vi "Function Generator.vi"(11 "Properties in":T1={"Schedule"=0, "Value"=0.0, "Start Value"=0.0, "End Value"=0.0, "Min Value"=0.0, "Max Value"=0.0, "Duty Cycle (%)"=0.0, "Speed Signal Type"=2, "Cycle Number"=0.0, "Phase (degrees)"=0.0} {"Schedule" items=["Constant", "Ramp", "Fn. Generator", "Formula"]; "Speed Signal Type" items=["Sine Wave", "Triangle Wave", "Square Wave", "Sawtooth Wave"]}) -> (2 "Properties out":T1={"Schedule"=0, "Value"=0.0, "Start Value"=0.0, "End Value"=0.0, "Min Value"=1.0, "Max Value"=3.0, "Duty Cycle (%)"=56.0, "Speed Signal Type"=0, "Cycle Number"=3.0, "Phase (degrees)"=90.0} {"Schedule" items=["Constant", "Ramp", "Fn. Generator", "Formula"]; "Speed Signal Type" items=["Sine Wave", "Triangle Wave", "Square Wave", "Sawtooth Wave"]}, 3 "Cancelled?":bool)   [LabVIEW 2013]
doc: "Use this template to create a dialog box with event handling."
uses:
  <vilib>/measure/NI_MABase.lvlib
panel:
  in  "Samples (testing)":dbl=1000.0
  out "Signal":dbl[](graph)=[3.0, 2.999822352380809, 2.999289472640589, 2.998401550108975, 2.997158900260614, 2.99556196460308, 2.9936113105200084, 2.991307631069507, 2.988651744737914, 2.9856445951489983, 2.982287250728689, 2.9785809043254723, 2.9745268727865772, 2.970126596490106, 2.965381638833274, 2.960293685676943, 2.954864544746643, 2.9490961449902944, 2.9429905358928643, 2.9365498867481925, 2.9297764858882513, 2.922672739870115, 2.9152411726209175, 2.907484424541117, 2.899405251566371, 2.891006524188368, 2.882291226434953, 2.87326245480992, 2.863923417192835, 2.854277431699295, 2.844327925502015, 2.834078433613171, 2.8235325976284273, 2.812694164433094, 2.8015669848708766, 2.79015501237569, 2.778462301567023, 2.76649300680935, 2.754251380736104, 2.741741772738739, 2.7289686274214113, 2.715936483021831, 2.7026499697988493, 2.6891138083873485, 2.6753328081210244, 2.661311865323652, 2.6470559615694444, 2.6325701619131245, 2.617859613090334, 2.602929541689025, 2.587785252292473, 2.572432125594591, 2.556875616488188, 2.5411212521268762, 2.525174629961296, 2.5090414157503713, 2.4927273415482913, 2.4762382036679393, 2.459579860621488, 2.4427582310389018, 2.425779291565073, 2.408649074736349, 2.3913736668372025, 2.3739592057378007, 2.3564118787132506, 2.3387379202452916, 2.3209436098072094, 2.3030352696327743, 2.285019262469976, 2.2669019893203757, 2.248689887164855, 2.2303894266765907, 2.212007109922055, 2.1935494680508603, 2.175023058975276, 2.156434465040231, 2.137790290684638, 2.11909716009487, 2.100361714851215, 2.0815906115681577, 2.0627905195293135, 2.0439681183178653, 2.0251300954433376, 2.0062831439655593, 1.9874339601166475, 1.968589240921872, 1.9497556818202306, 1.9309399742855944, 1.912148803449257, 1.8933888457247403, 1.874666766435696, 1.855989217447748, 1.8373628348051165, 1.8187942363728629, 1.800290019485593, 1.7818567586034577, 1.7635010029762754, 1.745229274316618, 1.727048064482675, 1.7089638331717283, 1.6909830056250528, 1.6731119703450577, 1.6553570768254833, 1.6377246332954545, 1.6202209044781992, 1.6028521093652195, 1.5856244190067161, 1.5685439543190411, 1.551616783909968, 1.5348489219225419, 1.518246325898285, 1.5018148946605094, 1.4855604662184938, 1.4694888156932662, 1.4536056532657313, 1.4379166221478696, 1.4224272965777327, 1.407143179838941, 1.392069702305395, 1.3772122195118879, 1.3625760102513107, 1.3481662746991216, 1.3339881325657488, 1.320046621277581, 1.3063466941871953, 1.2928932188134528, 1.2796909751120933, 1.2667446537774403, 1.2540588545758182, 1.2416380847112785, 1.229486757224211, 1.217609189423412, 1.2060096013521648, 1.1946921142888782, 1.1836607492828162, 1.1729194257254383, 1.1624719599578586, 1.152322063914917, 1.142473343806348, 1.1329292988355102, 1.1236933199561365, 1.114768688667545, 1.1061585758487364, 1.0978660406317973, 1.0898940293150043, 1.082245374316019, 1.074922793165542, 1.0679288875417892, 1.061266142346126, 1.0549369248201954, 1.0489434837048466, 1.04328794844117, 1.0379723284139142, 1.0329985122375653, 1.0283682670853262, 1.024083238061253, 1.0201449476157534, 1.0165547950046707, 1.013314055792132, 1.0104238813973492, 1.0078852986855225, 1.0056992096030013, 1.0038663908568277, 1.0023874936387749, 1.0012630433939829, 1.0004934396342686, 1.0000789557961842, 1.000019739143863, 1.0003158107167003, 1.0009670653218754, 1.0019732715717287, 1.0033340719659702, 1.0050489830187002, 1.0071173954301864, 1.009538574303349, 1.0123116594048622, 1.0154356654707948, 1.018909482556666, 1.0227318764318067, 1.0269014890178734, 1.031416838871369, 1.0362763217099902, 1.0414782109826244, 1.047020658482781, 1.0529016950052559, 1.0591192310457744, 1.065671057543388, 1.0725548466653385, 1.0797681526341298, 1.0873084125964971, 1.0951729475339806, 1.103358963214764, 1.1118635511864556, 1.1206836898094434, 1.1298162453304745, 1.139257972996056, 1.1490055182053083, 1.1590554177018304, 1.1694041008041873, 1.1800478906745473, 1.1909830056250525, 1.2022055604614286, 1.2137115678633812, 1.2254969398012658, 1.2375574889885521, 1.24988893036954, 1.2624868826418263, 1.2753468698129529, 1.2884643227907149, 1.3018345810065268, 1.3154528940713113, 1.3293144234632794, 1.3434142442470436, 1.3577473468234151, 1.3723086387092995, 1.387092946347023, 1.4020950169424813, 1.4173095203314234, 1.4327310508732436, 1.4483541293715692, 1.4641732050210035, 1.48018265737929, 1.4963767983642393, 1.5127498742746672, 1.5292960678346674, 1.5460095002604528, 1.5628842333490671, 1.5799142715881933, 1.5970935642863373, 1.6144160077226029, 1.631875447315322, 1.6494656798087406, 1.6671804554770133, 1.6850134803446948, 1.702958418422965, 1.7210088939607702, 1.739158493710103, 1.757400769204592, 1.7757292390506187, 1.7941373912301182, 1.8126186854142752, 1.8311665552872656, 1.8497744108792429, 1.868435640907717, 1.8871436151265182, 1.9058916866814852, 1.9246731944720672, 1.9434814655179748, 1.9623098173300653, 1.9811515602845913, 1.9999999999999998, 2.018848439715408, 2.0376901826699343, 2.056518534482024, 2.0753268055279324, 2.0941083133185137, 2.1128563848734814, 2.131564359092282, 2.150225589120757, 2.1688334447127335, 2.1873813145857244, 2.205862608769881, 2.224270760949381, 2.242599230795407, 2.2608415062898968, 2.2789911060392285, 2.2970415815770346, 2.3149865196553043, 2.3328195445229865, 2.3505343201912585, 2.3681245526846775, 2.385583992277396, 2.4029064357136622, 2.420085728411806, 2.4371157666509324, 2.4539904997395463, 2.4707039321653324, 2.487250125725332, 2.5036232016357607, 2.519817342620709, 2.535826794978996, 2.5516458706284295, 2.567268949126756, 2.5826904796685755, 2.5979049830575187, 2.612907053652976, 2.6276913612907, 2.642252653176584, 2.656585755752956, 2.6706855765367195, 2.6845471059286883, 2.6981654189934723, 2.7115356772092847, 2.724653130187046, 2.7375131173581737, 2.750111069630459, 2.7624425110114474, 2.7745030601987333, 2.7862884321366184, 2.7977944395385705, 2.809016994374947, 2.819952109325452, 2.8305958991958122, 2.8409445822981687, 2.8509944817946913, 2.860742027003943, 2.870183754669525, 2.879316310190556, 2.888136448813544, 2.8966410367852355, 2.904827052466019, 2.9126915874035024, 2.92023184736587, 2.927445153334661, 2.9343289424566117, 2.9408807689542256, 2.9470983049947437, 2.952979341517219, 2.9585217890173756, 2.96372367829001, 2.9685831611286306, 2.9730985109821266, 2.977268123568193, 2.9810905174433344, 2.984564334529205, 2.9876883405951378, 2.990461425696651, 2.9928826045698136, 2.9949510169813, 2.99666592803403, 2.9980267284282713, 2.999032934678125, 2.9996841892832995, 2.9999802608561374, 2.999921044203816, 2.999506560365732, 2.998736956606017, 2.9976125063612256, 2.996133609143172, 2.9943007903969994, 2.9921147013144775, 2.9895761186026513, 2.986685944207868, 2.9834452049953297, 2.9798550523842464, 2.9759167619387474, 2.9716317329146738, 2.9670014877624356, 2.9620276715860854, 2.9567120515588305, 2.951056516295153, 2.9450630751798053, 2.9387338576538737, 2.9320711124582113, 2.925077206834458, 2.9177546256839815, 2.910105970684995, 2.902133959368203, 2.8938414241512636, 2.8852313113324555, 2.8763066800438635, 2.8670707011644905, 2.8575266561936523, 2.8476779360850837, 2.8375280400421414, 2.827080574274562, 2.816339250717184, 2.805307885711122, 2.793990398647835, 2.7823908105765884, 2.770513242775789, 2.7583619152887224, 2.745941145424182, 2.7332553462225606, 2.720309024887907, 2.707106781186548, 2.693653305812805, 2.67995337872242, 2.6660118674342517, 2.6518337253008792, 2.6374239897486897, 2.622787780488113, 2.6079302976946055, 2.59285682016106, 2.577572703422268, 2.5620833778521312, 2.546394346734269, 2.530511184306735, 2.5144395337815064, 2.4981851053394917, 2.4817536741017157, 2.465151078077459, 2.4483832160900327, 2.4314560456809597, 2.4143755809932843, 2.3971478906347814, 2.3797790955218012, 2.362275366704546, 2.344642923174517, 2.3268880296549432, 2.309016994374948, 2.2910361668282726, 2.2729519355173258, 2.254770725683383, 2.236498997023725, 2.218143241396543, 2.1997099805144074, 2.1812057636271382, 2.162637165194884, 2.144010782552253, 2.1253332335643047, 2.1066111542752606, 2.0878511965507434, 2.0690600257144065, 2.05024431817977, 2.031410759078129, 2.012566039883353, 1.9937168560344418, 1.974869904556663, 1.9560318816821358, 1.937209480470687, 1.9184093884318432, 1.8996382851487856, 1.8809028399051309, 1.8622097093153624, 1.8435655349597697, 1.8249769410247245, 1.8064505319491404, 1.7879928900779458, 1.7696105733234102, 1.7513101128351458, 1.7330980106796252, 1.7149807375300243, 1.6969647303672266, 1.679056390192791, 1.6612620797547093, 1.6435881212867498, 1.6260407942622002, 1.6086263331627981, 1.5913509252636515, 1.5742207084349278, 1.5572417689610991, 1.5404201393785126, 1.5237617963320613, 1.5072726584517089, 1.4909585842496291, 1.4748253700387048, 1.4588787478731247, 1.4431243835118126, 1.4275678744054094, 1.4122147477075275, 1.3970704583109756, 1.3821403869096662, 1.367429838086876, 1.3529440384305562, 1.3386881346763486, 1.324667191878976, 1.310886191612652, 1.2973500302011514, 1.2840635169781691, 1.2710313725785891, 1.258258227261261, 1.2457486192638967, 1.2335069931906504, 1.221537698432977, 1.2098449876243098, 1.1984330151291238, 1.1873058355669062, 1.176467402371573, 1.165921566386829, 1.1556720744979856, 1.1457225683007048, 1.1360765828071653, 1.1267375451900798, 1.1177087735650473, 1.1089934758116322, 1.1005947484336294, 1.092515575458883, 1.084758827379083, 1.0773272601298851, 1.070223514111749, 1.0634501132518075, 1.0570094641071361, 1.0509038550097052, 1.0451354552533574, 1.0397063143230567, 1.0346183611667266, 1.029873403509894, 1.0254731272134232, 1.0214190956745277, 1.0177127492713116, 1.0143554048510017, 1.0113482552620865, 1.0086923689304932, 1.006388689479992, 1.0044380353969196, 1.0028410997393864, 1.0015984498910246, 1.000710527359411, 1.0001776476191906, 1.0000000000000002, 1.0001776476191906, 1.000710527359411, 1.0015984498910246, 1.0028410997393862, 1.0044380353969196, 1.0063886894799916, 1.0086923689304932, 1.011348255262086, 1.0143554048510017, 1.0177127492713114, 1.0214190956745275, 1.0254731272134228, 1.0298734035098938, 1.0346183611667261, 1.0397063143230565, 1.045135455253357, 1.050903855009705, 1.0570094641071355, 1.063450113251807, 1.0702235141117487, 1.0773272601298847, 1.0847588273790825, 1.0925155754588824, 1.100594748433629, 1.1089934758116318, 1.1177087735650466, 1.1267375451900792, 1.1360765828071644, 1.1457225683007044, 1.1556720744979847, 1.1659215663868283, 1.1764674023715722, 1.1873058355669055, 1.198433015129123, 1.209844987624309, 1.2215376984329762, 1.2335069931906495, 1.2457486192638958, 1.2582582272612601, 1.2710313725785882, 1.284063516978168, 1.2973500302011503, 1.3108861916126509, 1.3246671918789752, 1.3386881346763473, 1.352944038430555, 1.3674298380868748, 1.3821403869096651, 1.3970704583109745, 1.4122147477075262, 1.4275678744054083, 1.4431243835118113, 1.4588787478731233, 1.4748253700387037, 1.4909585842496278, 1.5072726584517078, 1.5237617963320602, 1.5404201393785115, 1.5572417689610978, 1.5742207084349267, 1.5913509252636502, 1.608626333162797, 1.6260407942621988, 1.6435881212867485, 1.6612620797547077, 1.6790563901927897, 1.6969647303672253, 1.7149807375300232, 1.7330980106796237, 1.7513101128351445, 1.7696105733234087, 1.7879928900779447, 1.8064505319491388, 1.8249769410247232, 1.8435655349597684, 1.8622097093153611, 1.8809028399051295, 1.8996382851487843, 1.9184093884318416, 1.9372094804706859, 1.9560318816821343, 1.9748699045566618, 1.9937168560344403, 2.012566039883352, 2.0314107590781276, 2.050244318179769, 2.069060025714405, 2.0878511965507425, 2.1066111542752592, 2.1253332335643034, 2.1440107825522516, 2.162637165194883, 2.1812057636271365, 2.1997099805144065, 2.218143241396542, 2.236498997023724, 2.2547707256833815, 2.2729519355173244, 2.2910361668282713, 2.3090169943749466, 2.326888029654942, 2.3446429231745163, 2.362275366704545, 2.3797790955218003, 2.39714789063478, 2.4143755809932834, 2.4314560456809584, 2.448383216090032, 2.465151078077458, 2.4817536741017148, 2.4981851053394903, 2.514439533781506, 2.5305111843067336, 2.5463943467342687, 2.56208337785213, 2.577572703422267, 2.5928568201610585, 2.607930297694605, 2.622787780488112, 2.6374239897486893, 2.6518337253008784, 2.6660118674342512, 2.6799533787224186, 2.6936533058128047, 2.707106781186547, 2.7203090248879063, 2.7332553462225597, 2.7459411454241818, 2.758361915288721, 2.770513242775789, 2.7823908105765875, 2.793990398647835, 2.8053078857111213, 2.8163392507171836, 2.8270805742745617, 2.8375280400421414, 2.847677936085083, 2.8575266561936523, 2.86707070116449, 2.8763066800438635, 2.885231311332455, 2.8938414241512636, 2.9021339593682027, 2.9101059706849957, 2.917754625683981, 2.925077206834458, 2.932071112458211, 2.938733857653874, 2.945063075179805, 2.9510565162951536, 2.9567120515588305, 2.962027671586086, 2.967001487762435, 2.9716317329146738, 2.9759167619387474, 2.979855052384247, 2.9834452049953297, 2.986685944207868, 2.989576118602651, 2.9921147013144775, 2.994300790396999, 2.9961336091431723, 2.997612506361225, 2.9987369566060176, 2.999506560365732, 2.9999210442038162, 2.9999802608561374, 2.9996841892833, 2.999032934678125, 2.998026728428272, 2.99666592803403, 2.9949510169813003, 2.992882604569814, 2.9904614256966515, 2.987688340595138, 2.9845643345292054, 2.9810905174433344, 2.9772681235681935, 2.973098510982127, 2.9685831611286315, 2.9637236782900103, 2.958521789017376, 2.9529793415172194, 2.9470983049947446, 2.940880768954226, 2.934328942456612, 2.927445153334662, 2.9202318473658706, 2.9126915874035033, 2.90482705246602, 2.8966410367852364, 2.888136448813545, 2.879316310190557, 2.870183754669526, 2.8607420270039445, 2.850994481794692, 2.84094458229817, 2.830595899195813, 2.8199521093254534, 2.809016994374948, 2.797794439538572, 2.7862884321366197, 2.774503060198735, 2.7624425110114483, 2.7501110696304605, 2.7375131173581746, 2.724653130187048, 2.711535677209286, 2.6981654189934736, 2.684547105928689, 2.6706855765367212, 2.656585755752957, 2.6422526531765853, 2.627691361290701, 2.6129070536529775, 2.5979049830575196, 2.5826904796685772, 2.567268949126757, 2.5516458706284313, 2.5358267949789974, 2.5198173426207107, 2.5036232016357616, 2.4872501257253337, 2.4707039321653332, 2.453990499739548, 2.4371157666509338, 2.4200857284118076, 2.4029064357136636, 2.3855839922773976, 2.368124552684679, 2.3505343201912603, 2.3328195445229873, 2.314986519655306, 2.2970415815770355, 2.2789911060392303, 2.2608415062898977, 2.242599230795409, 2.224270760949382, 2.2058626087698827, 2.1873813145857257, 2.1688334447127353, 2.150225589120758, 2.131564359092284, 2.1128563848734827, 2.0941083133185154, 2.0753268055279337, 2.056518534482026, 2.0376901826699356, 2.0188484397154096, 2.000000000000001, 1.981151560284593, 1.9623098173300664, 1.9434814655179766, 1.924673194472068, 1.9058916866814868, 1.887143615126519, 1.8684356409077187, 1.8497744108792438, 1.8311665552872674, 1.8126186854142763, 1.7941373912301197, 1.7757292390506196, 1.7574007692045936, 1.739158493710104, 1.721008893960772, 1.7029584184229658, 1.6850134803446963, 1.6671804554770142, 1.649465679808742, 1.6318754473153227, 1.6144160077226044, 1.5970935642863382, 1.5799142715881946, 1.5628842333490678, 1.5460095002604541, 1.529296067834668, 1.5127498742746686, 1.4963767983642398, 1.4801826573792916, 1.4641732050210041, 1.4483541293715707, 1.4327310508732443, 1.417309520331425, 1.4020950169424817, 1.3870929463470243, 1.3723086387093002, 1.3577473468234165, 1.3434142442470443, 1.3293144234632808, 1.315452894071312, 1.3018345810065282, 1.2884643227907153, 1.275346869812954, 1.2624868826418267, 1.2498889303695413, 1.2375574889885526, 1.2254969398012667, 1.2137115678633816, 1.2022055604614295, 1.190983005625053, 1.1800478906745482, 1.1694041008041878, 1.1590554177018313, 1.1490055182053087, 1.1392579729960568, 1.1298162453304748, 1.120683689809444, 1.1118635511864559, 1.1033589632147645, 1.0951729475339809, 1.0873084125964976, 1.07976815263413, 1.072554846665339, 1.0656710575433883, 1.0591192310457749, 1.0529016950052559, 1.0470206584827815, 1.0414782109826244, 1.0362763217099904, 1.0314168388713691, 1.0269014890178734, 1.0227318764318067, 1.018909482556666, 1.0154356654707948, 1.0123116594048622, 1.009538574303349, 1.0071173954301862, 1.0050489830187, 1.0033340719659698, 1.0019732715717284, 1.000967065321875, 1.0003158107167, 1.0000197391438626, 1.0000789557961838, 1.0004934396342682, 1.0012630433939824, 1.0023874936387744, 1.0038663908568273, 1.0056992096030006, 1.007885298685522, 1.0104238813973485, 1.0133140557921316, 1.0165547950046698, 1.0201449476157527, 1.0240832380612521, 1.0283682670853258, 1.0329985122375644, 1.0379723284139137, 1.043287948441169, 1.048943483704846, 1.0549369248201945, 1.0612661423461254, 1.0679288875417883, 1.0749227931655416, 1.082245374316018, 1.089894029315004, 1.0978660406317964, 1.1061585758487356, 1.114768688667544, 1.1236933199561359, 1.132929298835509, 1.1424733438063472, 1.1523220639149159, 1.1624719599578577, 1.1729194257254374, 1.1836607492828155, 1.1946921142888773, 1.206009601352164, 1.2176091894234111, 1.22948675722421, 1.2416380847112771, 1.254058854575817, 1.266744653777439, 1.2796909751120922, 1.2928932188134517, 1.306346694187194, 1.3200466212775799, 1.3339881325657474, 1.3481662746991203, 1.3625760102513094, 1.3772122195118865, 1.3920697023053936, 1.4071431798389398, 1.4224272965777314, 1.4379166221478683, 1.45360565326573, 1.469488815693265, 1.4855604662184925, 1.501814894660508, 1.5182463258982837, 1.5348489219225407, 1.5516167839099666, 1.56854395431904, 1.5856244190067148, 1.6028521093652184, 1.6202209044781977, 1.6377246332954531, 1.6553570768254817, 1.6731119703450563, 1.6909830056250514, 1.708963833171727, 1.7270480644826736, 1.7452292743166167, 1.763501002976274, 1.7818567586034564, 1.8002900194855918, 1.8187942363728615, 1.8373628348051152, 1.8559892174477466, 1.8746667664356944, 1.8933888457247388, 1.9121488034492555, 1.930939974285593, 1.9497556818202293, 1.9685892409218704, 1.9874339601166462, 2.0062831439655575, 2.025130095443336, 2.0439681183178635, 2.062790519529312, 2.0815906115681564, 2.1003617148512137, 2.1190971600948685, 2.1377902906846367, 2.1564344650402294, 2.175023058975275, 2.193549468050859, 2.2120071099220535, 2.2303894266765893, 2.2486898871648537, 2.2669019893203743, 2.2850192624699748, 2.3030352696327725, 2.3209436098072085, 2.3387379202452903, 2.3564118787132498, 2.3739592057377994, 2.391373666837201, 2.408649074736348, 2.4257792915650715, 2.4427582310389004, 2.4595798606214867, 2.476238203667938, 2.4927273415482905, 2.50904141575037, 2.5251746299612945, 2.541121252126875, 2.556875616488187, 2.57243212559459, 2.5877852522924725, 2.602929541689024, 2.6178596130903333, 2.632570161913123, 2.6470559615694436, 2.661311865323651, 2.6753328081210235, 2.6891138083873476, 2.7026499697988484, 2.71593648302183, 2.728968627421411, 2.741741772738738, 2.754251380736103, 2.766493006809349, 2.778462301567023, 2.7901550123756893, 2.801566984870876, 2.8126941644330934, 2.823532597628427, 2.8340784336131706, 2.844327925502015, 2.8542774316992947, 2.863923417192835, 2.8732624548099195, 2.882291226434953, 2.8910065241883673, 2.899405251566371, 2.907484424541116, 2.9152411726209175, 2.922672739870114, 2.9297764858882513, 2.9365498867481916, 2.9429905358928643, 2.949096144990294, 2.954864544746643, 2.960293685676943, 2.965381638833274, 2.9701265964901054, 2.9745268727865772, 2.978580904325472, 2.982287250728689, 2.985644595148998, 2.988651744737914, 2.9913076310695064, 2.9936113105200084, 2.9955619646030796, 2.9971589002606143, 2.9984015501089747, 2.9992894726405894, 2.999822352380809]
  in  "Signal Type":u16(ring) items=["Sine Wave", "Triangle Wave", "Square Wave", "Sawtooth Wave"]
  in  "Phase (degrees)":dbl=90.0
  in  "Cycle Number":dbl=3.0
  in  "Square Wave\nDuty Cycle (%)":dbl=56.0
  in  "Max Value":dbl=3.0
  in  "Min Value":dbl=1.0
  in  "Cancel":bool
  in  "OK":bool
  # "Function Generator"
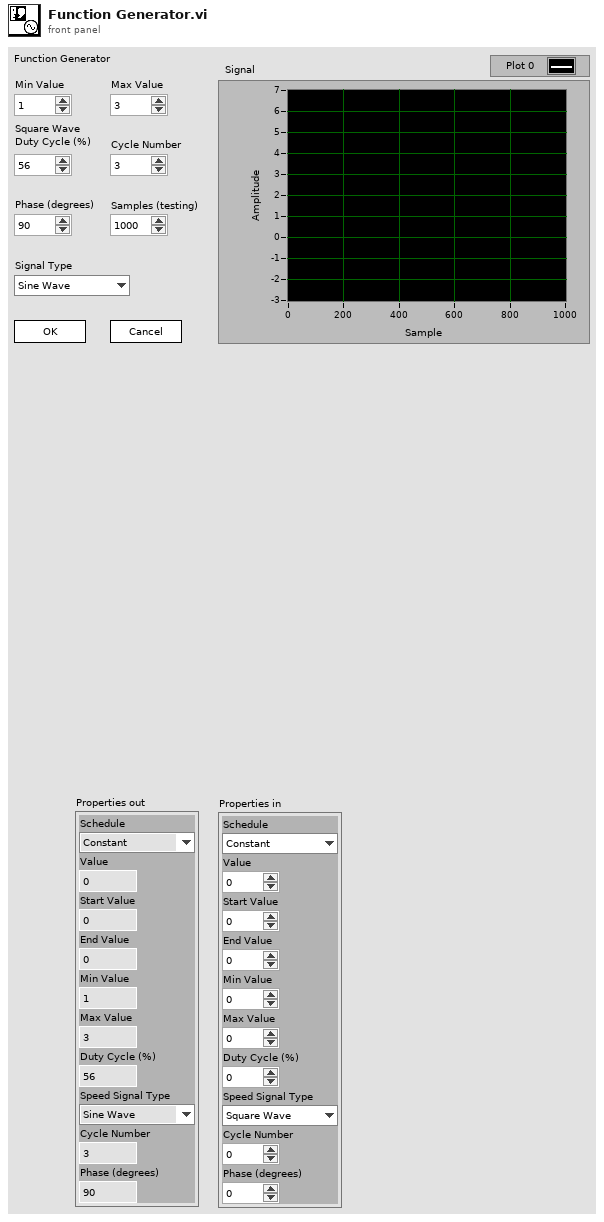
[diagram p1: front panel]
types:
  T1 = cluster{"Schedule":u16, "Value":dbl, "Start Value":dbl, "End Value":dbl, "Min Value":dbl, "Max Value":dbl, "Duty Cycle (%)":dbl, "Speed Signal Type":u16, "Cycle Number":dbl, "Phase (degrees)":dbl}
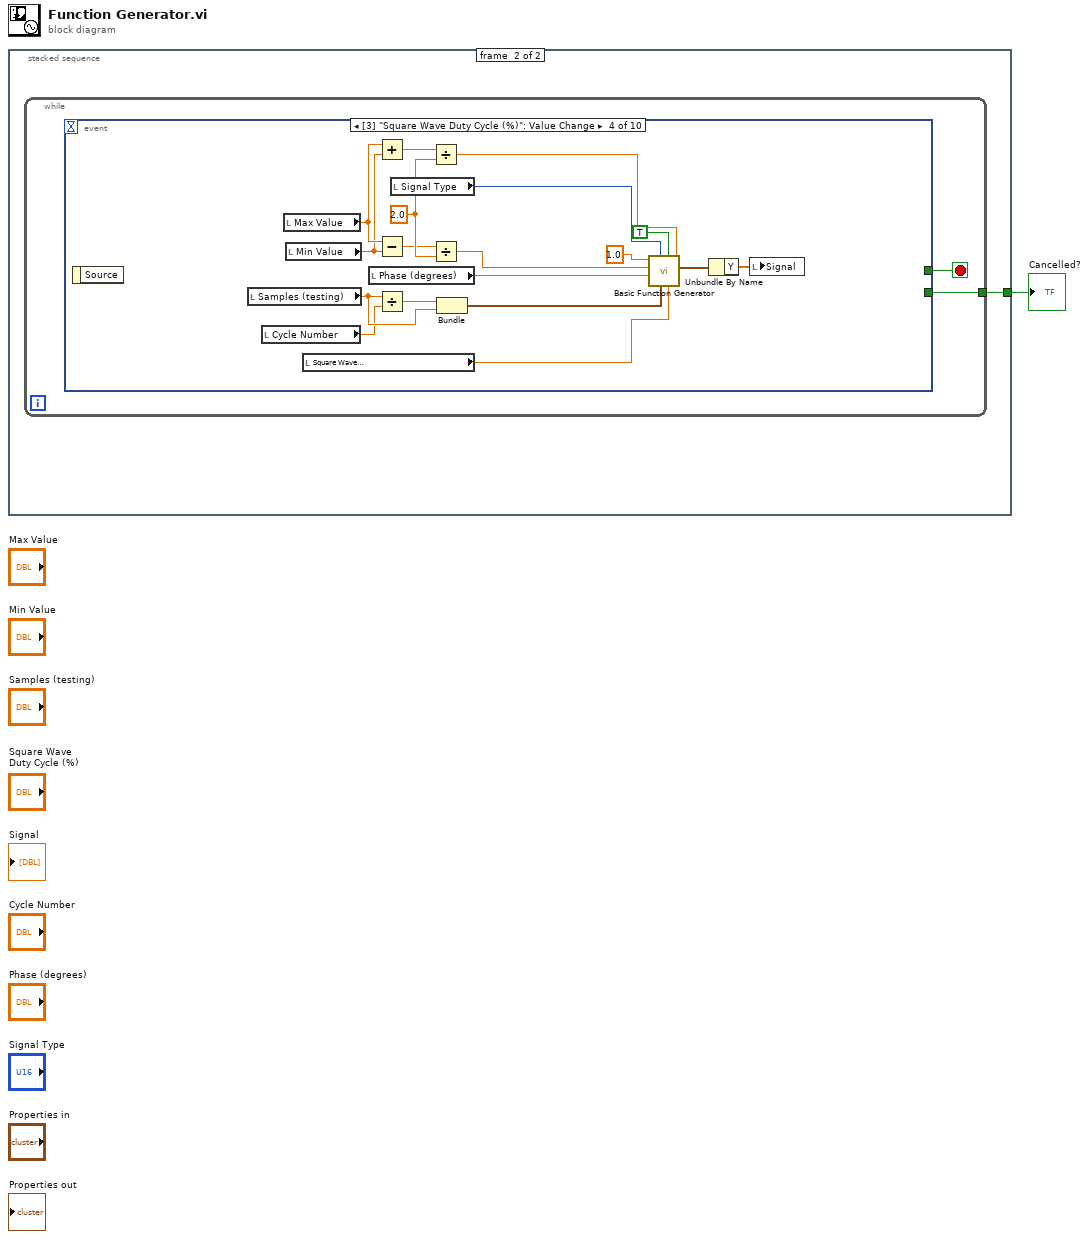
[diagram p0: block diagram]
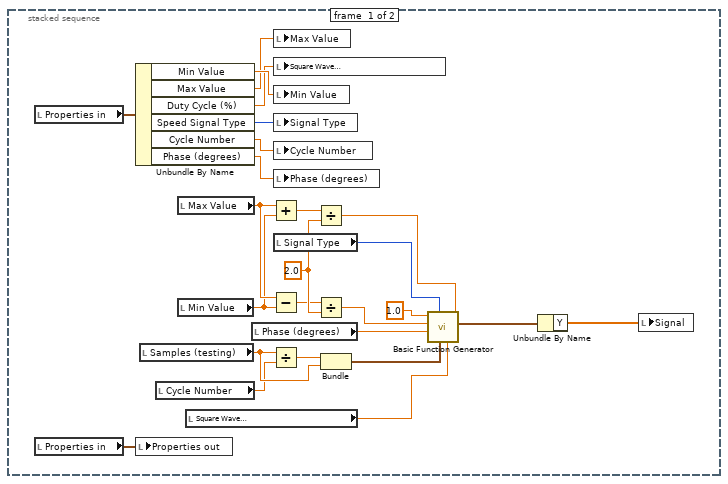
[diagram p2: hidden frame]
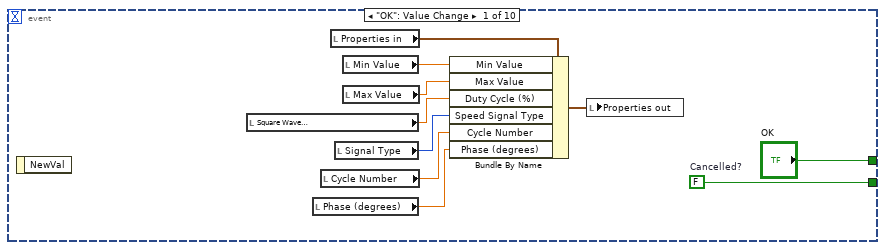
[diagram p3: hidden frame]
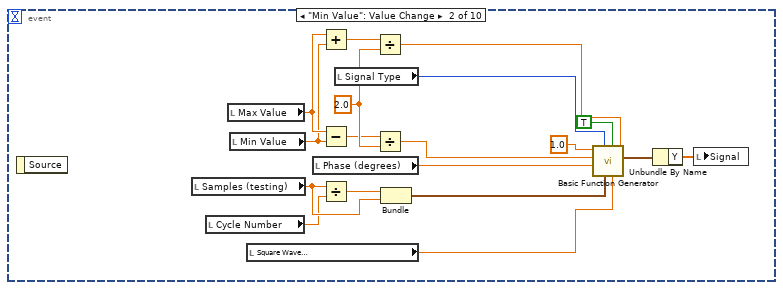
[diagram p4: hidden frame]
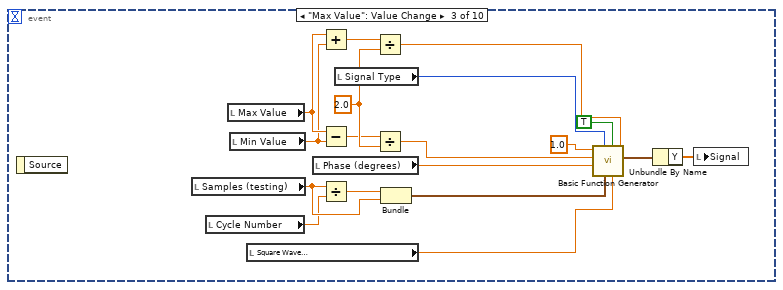
[diagram p5: hidden frame]
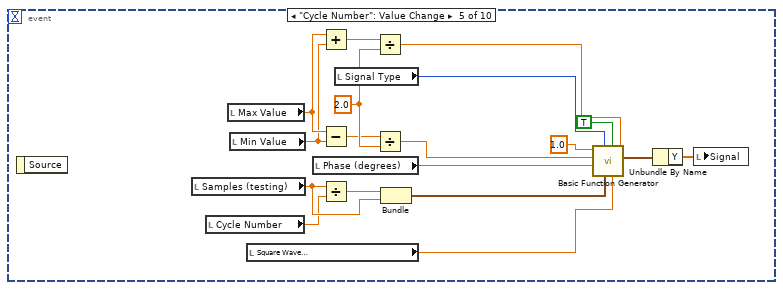
[diagram p6: hidden frame]
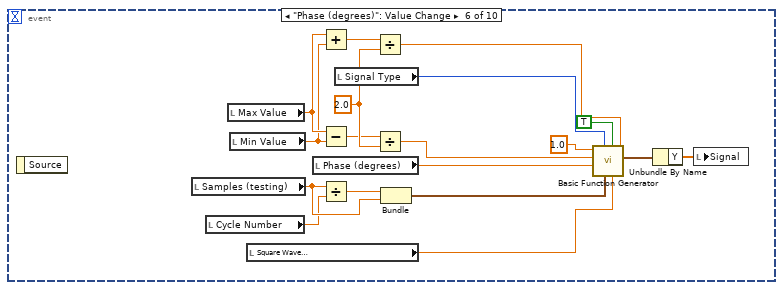
[diagram p7: hidden frame]
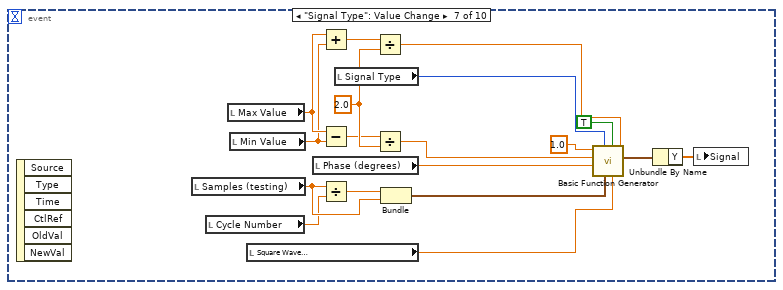
[diagram p8: hidden frame]
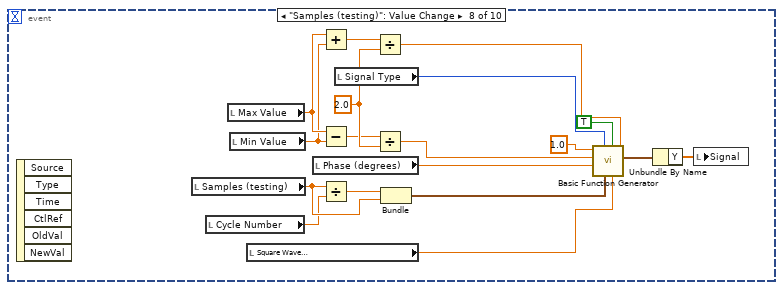
[diagram p9: hidden frame]
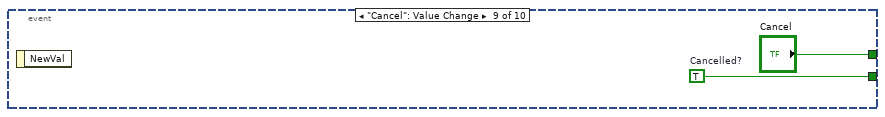
[diagram p10: hidden frame]
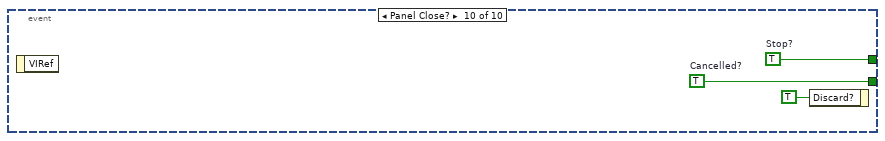
[diagram p11: hidden frame]
diagram:
  n1 = stacked-sequence {
    tunnel: [_ w27] -> w1
    frame #0 {
      w15 = 2.0 ("y")
      n2 = local read "Properties in"() -> (w26:T1)
      n3 = local read "Properties in"() -> (w2:T1)
      n4 = Unbundle By Name(w26) -> ("Min Value"=w25:dbl, "Max Value"=w24:dbl, "Duty Cycle (%)"=w23:dbl, "Speed Signal Type"=w22:u16, "Cycle Number"=w21:dbl, "Phase (degrees)"=w20:dbl)
      n5 = local write "Properties out"(w2) -> ()
      n6 = local read "Samples (testing)"() -> (w8:dbl)
      n7 = local read "Cycle Number"() -> (w7:dbl)
      n8 = local read "Max Value"() -> (w19:dbl)
      n9 = local read "Min Value"() -> (w6:dbl)
      n10 = local read "Square Wave\nDuty Cycle (%)"() -> (w4:dbl)
      n11 = local read "Phase (degrees)"() -> (w3:dbl)
      n12 = Add(x=w19, y=w6) -> (x+y=w12:dbl)
      n13 = Subtract(x=w19, y=w6) -> (x-y=w14:dbl)
      n14 = Divide(x=w8, y=w7) -> (x/y=w18:dbl)
      n15 = local write "Max Value"(w24) -> ()
      n16 = local write "Square Wave\nDuty Cycle (%)"(w23) -> ()
      n17 = local write "Min Value"(w25) -> ()
      n18 = local write "Signal Type"(w22) -> ()
      n19 = local write "Cycle Number"(w21) -> ()
      n20 = local write "Phase (degrees)"(w20) -> ()
      n21 = local read "Signal Type"() -> (w5:u16)
      n22 = Divide(x=w12, y=w15) -> (x/y=w13:dbl)
      n23 = Divide(x=w14, y=w15) -> (x/y=w16:dbl)
      n24 = Bundle(w18, "Samples (testing)"=w8) -> (w17:cluster{dbl, "Samples (testing)":dbl})  [unwired: 1 in]
      n25 = call <vilib>:"Basic Function Generator.vi"("offset"=w13, "square wave duty cycle (%)"=w4, "sampling info"=w17, "signal type"=w5, "phase"=w3, "amplitude"=w16, "frequency"=1.0) -> ("signal out"=w10:waveform(dbl))  [unwired: 2 in, 2 out]
      n26 = Unbundle By Name(w10) -> ("Y"=w9:dbl[])
      n27 = local write "Signal"(w9) -> ()
    }
    frame #1 {
      n28 = while {
        tunnel: [w28] -> w27
        stop <- w29 stop-if-true
        n29 = event shown="[3] \"Square Wave Duty Cycle (%)\": Value Change" {
          selector: _ -> [_ _ _ _ _ _ _ _ _ _]
          dyn-events: _ -> [_ _ _ _ _ _ _ _ _ _]
          timeout: _ -> [_ _ _ _ _ _ _ _ _ _]
          tunnel: ["OK" _ _ _ _ _ _ _ "Cancel" w169] -> w29
          tunnel: [w39 _ _ _ _ _ _ _ w167 w168] -> w28
          event "OK": Value Change {
            w39 = FALSE  # Cancelled?
            n30 = event-data() -> ()  [unwired: 1 in, 1 out]
            n31 = local read "Square Wave\nDuty Cycle (%)"() -> (w35:dbl)
            n32 = local read "Phase (degrees)"() -> (w32:dbl)
            n33 = local read "Cycle Number"() -> (w33:dbl)
            n34 = local read "Properties in"() -> (w31:T1)
            n35 = local read "Signal Type"() -> (w34:u16)
            n36 = local read "Min Value"() -> (w37:dbl)
            n37 = local read "Max Value"() -> (w36:dbl)
            n38 = Bundle By Name(cluster=w31, "Min Value"=w37, "Max Value"=w36, "Duty Cycle (%)"=w35, "Speed Signal Type"=w34, "Cycle Number"=w33, "Phase (degrees)"=w32) -> (w30:T1)
            n39 = local write "Properties out"(w30) -> ()
          }
          event "Min Value": Value Change {
            w54 = 2.0 ("y")
            n40 = event-data() -> ()  [unwired: 1 in, 1 out]
            n41 = local read "Samples (testing)"() -> (w47:dbl)
            n42 = local read "Cycle Number"() -> (w46:dbl)
            n43 = local read "Max Value"() -> (w45:dbl)
            n44 = local read "Min Value"() -> (w44:dbl)
            n45 = local read "Square Wave\nDuty Cycle (%)"() -> (w42:dbl)
            n46 = local read "Phase (degrees)"() -> (w41:dbl)
            n47 = Add(x=w45, y=w44) -> (x+y=w51:dbl)
            n48 = Subtract(x=w45, y=w44) -> (x-y=w53:dbl)
            n49 = Divide(x=w47, y=w46) -> (x/y=w57:dbl)
            n50 = local read "Signal Type"() -> (w43:u16)
            n51 = Divide(x=w51, y=w54) -> (x/y=w52:dbl)
            n52 = Divide(x=w53, y=w54) -> (x/y=w55:dbl)
            n53 = Bundle(w57, "Samples (testing)"=w47) -> (w56:cluster{dbl, "Samples (testing)":dbl})  [unwired: 1 in]
            n54 = call <vilib>:"Basic Function Generator.vi"("offset"=w52, "square wave duty cycle (%)"=w42, "reset signal"=TRUE, "sampling info"=w56, "signal type"=w43, "phase"=w41, "amplitude"=w55, "frequency"=1.0) -> ("signal out"=w49:waveform(dbl))  [unwired: 1 in, 2 out]
            n55 = Unbundle By Name(w49) -> ("Y"=w48:dbl[])
            n56 = local write "Signal"(w48) -> ()
          }
          event "Max Value": Value Change {
            w72 = 2.0 ("y")
            n57 = event-data() -> ()  [unwired: 1 in, 1 out]
            n58 = local read "Samples (testing)"() -> (w65:dbl)
            n59 = local read "Cycle Number"() -> (w64:dbl)
            n60 = local read "Max Value"() -> (w63:dbl)
            n61 = local read "Min Value"() -> (w62:dbl)
            n62 = local read "Square Wave\nDuty Cycle (%)"() -> (w60:dbl)
            n63 = local read "Phase (degrees)"() -> (w59:dbl)
            n64 = Add(x=w63, y=w62) -> (x+y=w69:dbl)
            n65 = Subtract(x=w63, y=w62) -> (x-y=w71:dbl)
            n66 = Divide(x=w65, y=w64) -> (x/y=w75:dbl)
            n67 = local read "Signal Type"() -> (w61:u16)
            n68 = Divide(x=w69, y=w72) -> (x/y=w70:dbl)
            n69 = Divide(x=w71, y=w72) -> (x/y=w73:dbl)
            n70 = Bundle(w75, "Samples (testing)"=w65) -> (w74:cluster{dbl, "Samples (testing)":dbl})  [unwired: 1 in]
            n71 = call <vilib>:"Basic Function Generator.vi"("offset"=w70, "square wave duty cycle (%)"=w60, "reset signal"=TRUE, "sampling info"=w74, "signal type"=w61, "phase"=w59, "amplitude"=w73, "frequency"=1.0) -> ("signal out"=w67:waveform(dbl))  [unwired: 1 in, 2 out]
            n72 = Unbundle By Name(w67) -> ("Y"=w66:dbl[])
            n73 = local write "Signal"(w66) -> ()
          }
          event "Square Wave\nDuty Cycle (%)": Value Change {
            w90 = 2.0 ("y")
            n74 = event-data() -> ()  [unwired: 1 in, 1 out]
            n75 = local read "Samples (testing)"() -> (w83:dbl)
            n76 = local read "Cycle Number"() -> (w82:dbl)
            n77 = local read "Max Value"() -> (w81:dbl)
            n78 = local read "Min Value"() -> (w80:dbl)
            n79 = local read "Square Wave\nDuty Cycle (%)"() -> (w78:dbl)
            n80 = local read "Phase (degrees)"() -> (w77:dbl)
            n81 = Add(x=w81, y=w80) -> (x+y=w87:dbl)
            n82 = Subtract(x=w81, y=w80) -> (x-y=w89:dbl)
            n83 = Divide(x=w83, y=w82) -> (x/y=w93:dbl)
            n84 = local read "Signal Type"() -> (w79:u16)
            n85 = Divide(x=w87, y=w90) -> (x/y=w88:dbl)
            n86 = Divide(x=w89, y=w90) -> (x/y=w91:dbl)
            n87 = Bundle(w93, "Samples (testing)"=w83) -> (w92:cluster{dbl, "Samples (testing)":dbl})  [unwired: 1 in]
            n88 = call <vilib>:"Basic Function Generator.vi"("offset"=w88, "square wave duty cycle (%)"=w78, "reset signal"=TRUE, "sampling info"=w92, "signal type"=w79, "phase"=w77, "amplitude"=w91, "frequency"=1.0) -> ("signal out"=w85:waveform(dbl))  [unwired: 1 in, 2 out]
            n89 = Unbundle By Name(w85) -> ("Y"=w84:dbl[])
            n90 = local write "Signal"(w84) -> ()
          }
          event "Cycle Number": Value Change {
            w108 = 2.0 ("y")
            n91 = event-data() -> ()  [unwired: 1 in, 1 out]
            n92 = local read "Samples (testing)"() -> (w101:dbl)
            n93 = local read "Cycle Number"() -> (w100:dbl)
            n94 = local read "Max Value"() -> (w99:dbl)
            n95 = local read "Min Value"() -> (w98:dbl)
            n96 = local read "Square Wave\nDuty Cycle (%)"() -> (w96:dbl)
            n97 = local read "Phase (degrees)"() -> (w95:dbl)
            n98 = Add(x=w99, y=w98) -> (x+y=w105:dbl)
            n99 = Subtract(x=w99, y=w98) -> (x-y=w107:dbl)
            n100 = Divide(x=w101, y=w100) -> (x/y=w111:dbl)
            n101 = local read "Signal Type"() -> (w97:u16)
            n102 = Divide(x=w105, y=w108) -> (x/y=w106:dbl)
            n103 = Divide(x=w107, y=w108) -> (x/y=w109:dbl)
            n104 = Bundle(w111, "Samples (testing)"=w101) -> (w110:cluster{dbl, "Samples (testing)":dbl})  [unwired: 1 in]
            n105 = call <vilib>:"Basic Function Generator.vi"("offset"=w106, "square wave duty cycle (%)"=w96, "reset signal"=TRUE, "sampling info"=w110, "signal type"=w97, "phase"=w95, "amplitude"=w109, "frequency"=1.0) -> ("signal out"=w103:waveform(dbl))  [unwired: 1 in, 2 out]
            n106 = Unbundle By Name(w103) -> ("Y"=w102:dbl[])
            n107 = local write "Signal"(w102) -> ()
          }
          event "Phase (degrees)": Value Change {
            w126 = 2.0 ("y")
            n108 = event-data() -> ()  [unwired: 1 in, 1 out]
            n109 = local read "Samples (testing)"() -> (w119:dbl)
            n110 = local read "Cycle Number"() -> (w118:dbl)
            n111 = local read "Max Value"() -> (w117:dbl)
            n112 = local read "Min Value"() -> (w116:dbl)
            n113 = local read "Square Wave\nDuty Cycle (%)"() -> (w114:dbl)
            n114 = local read "Phase (degrees)"() -> (w113:dbl)
            n115 = Add(x=w117, y=w116) -> (x+y=w123:dbl)
            n116 = Subtract(x=w117, y=w116) -> (x-y=w125:dbl)
            n117 = Divide(x=w119, y=w118) -> (x/y=w129:dbl)
            n118 = local read "Signal Type"() -> (w115:u16)
            n119 = Divide(x=w123, y=w126) -> (x/y=w124:dbl)
            n120 = Divide(x=w125, y=w126) -> (x/y=w127:dbl)
            n121 = Bundle(w129, "Samples (testing)"=w119) -> (w128:cluster{dbl, "Samples (testing)":dbl})  [unwired: 1 in]
            n122 = call <vilib>:"Basic Function Generator.vi"("offset"=w124, "square wave duty cycle (%)"=w114, "reset signal"=TRUE, "sampling info"=w128, "signal type"=w115, "phase"=w113, "amplitude"=w127, "frequency"=1.0) -> ("signal out"=w121:waveform(dbl))  [unwired: 1 in, 2 out]
            n123 = Unbundle By Name(w121) -> ("Y"=w120:dbl[])
            n124 = local write "Signal"(w120) -> ()
          }
          event "Signal Type": Value Change {
            w144 = 2.0 ("y")
            n125 = event-data() -> ()  [unwired: 1 in, 6 out]
            n126 = local read "Samples (testing)"() -> (w137:dbl)
            n127 = local read "Cycle Number"() -> (w136:dbl)
            n128 = local read "Max Value"() -> (w135:dbl)
            n129 = local read "Min Value"() -> (w134:dbl)
            n130 = local read "Square Wave\nDuty Cycle (%)"() -> (w132:dbl)
            n131 = local read "Phase (degrees)"() -> (w131:dbl)
            n132 = Add(x=w135, y=w134) -> (x+y=w141:dbl)
            n133 = Subtract(x=w135, y=w134) -> (x-y=w143:dbl)
            n134 = Divide(x=w137, y=w136) -> (x/y=w147:dbl)
            n135 = local read "Signal Type"() -> (w133:u16)
            n136 = Divide(x=w141, y=w144) -> (x/y=w142:dbl)
            n137 = Divide(x=w143, y=w144) -> (x/y=w145:dbl)
            n138 = Bundle(w147, "Samples (testing)"=w137) -> (w146:cluster{dbl, "Samples (testing)":dbl})  [unwired: 1 in]
            n139 = call <vilib>:"Basic Function Generator.vi"("offset"=w142, "square wave duty cycle (%)"=w132, "reset signal"=TRUE, "sampling info"=w146, "signal type"=w133, "phase"=w131, "amplitude"=w145, "frequency"=1.0) -> ("signal out"=w139:waveform(dbl))  [unwired: 1 in, 2 out]
            n140 = Unbundle By Name(w139) -> ("Y"=w138:dbl[])
            n141 = local write "Signal"(w138) -> ()
          }
          event "Samples (testing)": Value Change {
            w162 = 2.0 ("y")
            n142 = event-data() -> ()  [unwired: 1 in, 6 out]
            n143 = local read "Samples (testing)"() -> (w155:dbl)
            n144 = local read "Cycle Number"() -> (w154:dbl)
            n145 = local read "Max Value"() -> (w153:dbl)
            n146 = local read "Min Value"() -> (w152:dbl)
            n147 = local read "Square Wave\nDuty Cycle (%)"() -> (w150:dbl)
            n148 = local read "Phase (degrees)"() -> (w149:dbl)
            n149 = Add(x=w153, y=w152) -> (x+y=w159:dbl)
            n150 = Subtract(x=w153, y=w152) -> (x-y=w161:dbl)
            n151 = Divide(x=w155, y=w154) -> (x/y=w165:dbl)
            n152 = local read "Signal Type"() -> (w151:u16)
            n153 = Divide(x=w159, y=w162) -> (x/y=w160:dbl)
            n154 = Divide(x=w161, y=w162) -> (x/y=w163:dbl)
            n155 = Bundle(w165, "Samples (testing)"=w155) -> (w164:cluster{dbl, "Samples (testing)":dbl})  [unwired: 1 in]
            n156 = call <vilib>:"Basic Function Generator.vi"("offset"=w160, "square wave duty cycle (%)"=w150, "reset signal"=TRUE, "sampling info"=w164, "signal type"=w151, "phase"=w149, "amplitude"=w163, "frequency"=1.0) -> ("signal out"=w157:waveform(dbl))  [unwired: 1 in, 2 out]
            n157 = Unbundle By Name(w157) -> ("Y"=w156:dbl[])
            n158 = local write "Signal"(w156) -> ()
          }
          event "Cancel": Value Change {
            w167 = TRUE  # Cancelled?
            n159 = event-data() -> ()  [unwired: 1 in, 1 out]
          }
          event Panel Close? {
            w168 = TRUE  # Cancelled?
            w169 = TRUE  # Stop?
            n160 = event-data() -> ()  [unwired: 1 in, 1 out]
            n161 = event-data("Discard?"=TRUE) -> ()  [unwired: 1 in, 1 out]
          }
        }
      }
    }
  }
  "Cancelled?" <- w1
